vi "Get Selected UID.vi"() -> ()   [LabVIEW 2019]
panel:
  out "UID":i32
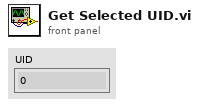
[diagram p1: front panel]
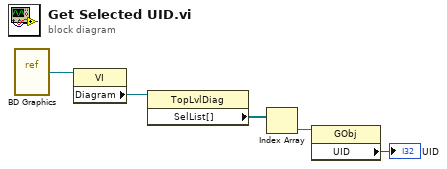
[diagram p0: block diagram]
diagram:
  n1 = vi-ref "BD Graphics.vi"() -> (w5:refnum<vi>)
  n2 = property class="VI"(reference=w5) -> ("Diagram"=w4:refnum<vi>)  [unwired: 1 in, 2 out]
  n3 = property class="TopLvlDiag"(reference=w4) -> ("SelList[]"=w3:refnum<vi>[])  [unwired: 1 in, 2 out]
  n4 = Index Array(array=w3) -> (element=w2:refnum<vi>)  [unwired: 1 in]
  n5 = property class="GObj"(reference=w2) -> ("UID"=→"UID":i32)  [unwired: 1 in, 2 out]
